vi "save channel config file.vi"(10 "Array":T1[](array[typedef]), 11 "file path":path) -> (3 "path":path)   [LabVIEW 2018]
uses:
  type defs/channelControl.ctl
  RT/Type Defs/channelScalingTypes.ctl
  RT/Type Defs/scalingMethods.ctl
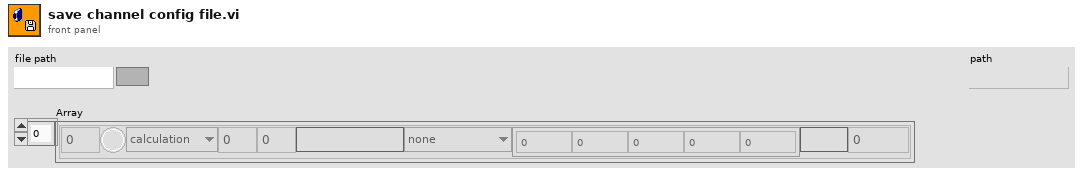
[diagram p1: front panel]
types:
  T1 = typedef "channelControl.ctl" = cluster{"index":u16, "active":bool, "channelType":T2, "module":u16, "terminal":u16, "channelName":string, "scalingMethod":T3, "scalingParameters":dbl[], "scaledUnits":string, "tempOffset":dbl}
  T2 = typedef "channelScalingTypes.ctl" = enum16{"calculation", "measurement", "scanivalve", "output", "digital"}
  T3 = typedef "scalingMethods.ctl" = enum16{"none", "linear", "thermocouple", "polynomial", "encoder", "RTD"}
  T4 = enum16{"open", "replace", "create", "open or create", "replace or create", "replace or create with confirmation"}
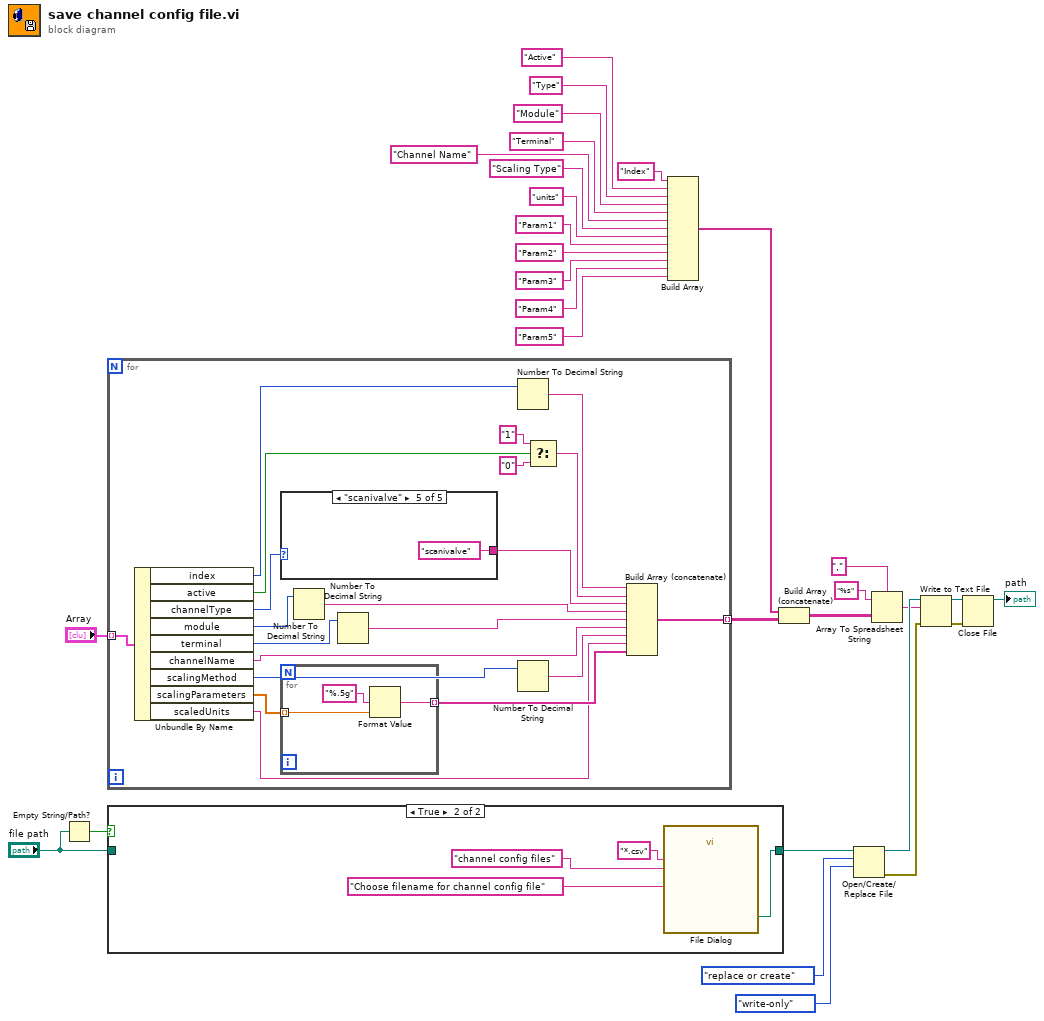
[diagram p0: block diagram]
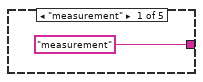
[diagram p3: hidden frame]
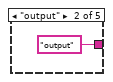
[diagram p4: hidden frame]
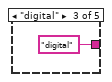
[diagram p5: hidden frame]
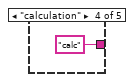
[diagram p6: hidden frame]
diagram:
  n1 = Empty String/Path?(string/path="file path") -> (empty?=w4:bool)
  n2 = for {
    tunnel: "Array" -> [w50] mode=indexing
    tunnel: [w38] -> w19 mode=indexing
    n3 = Unbundle By Name(w50) -> ("index"=w49:u16, "active"=w46:bool, "channelType"=w45:T2, "module"=w34:u16, "terminal"=w33:u16, "channelName"=w39:string, "scalingMethod"=w44:T3, "scalingParameters"=w43:dbl[], "scaledUnits"=w35:string)
    n4 = case shown="\"scanivalve\"" w45 {
      tunnel: ["measurement" ("f") "output" ("f") "digital" ("f") "calc" ("f") "scanivalve" ("f")] -> w40
      frame "measurement" {
      }
      frame "output" {
      }
      frame "digital" {
      }
      frame "calculation" {
      }
      frame "scanivalve" {
      }
    }
    n5 = for {
      tunnel: w43 -> [w53] mode=indexing
      tunnel: [w51] -> w37 mode=indexing
      n6 = Format Value(format string="%.5g", value (0)=w53) -> (output string=w51:string)  [unwired: 1 in]
    }
    n7 = Number To Decimal String(number=w34) -> (decimal integer string=w32:string)  [unwired: 1 in]
    n8 = Number To Decimal String(number=w33) -> (decimal integer string=w31:string)  [unwired: 1 in]
    n9 = Number To Decimal String(number=w49) -> (decimal integer string=w42:string)  [unwired: 1 in]
    n10 = Number To Decimal String(number=w44) -> (decimal integer string=w36:string)  [unwired: 1 in]
    n11 = Select(t="1", s=w46, f="0") -> (s? t:f=w41:string)
    n12 = Build Array (concatenate)(w42, w41, w40, w32, w31, w39, w36, w35, w37) -> (w38:string[])
  }
  n13 = case shown="True" w4 {
    tunnel: [w59 w62] -> w2
    tunnel: "file path" -> [w59 _]
    frame False {
    }
    frame True {
      n14 = call "File Dialog"("prompt"="Choose filename for channel config file", "pattern (all files)"="*.csv" ("pattern label"), "pattern label"="channel config files") -> ("selected path"=w62:path)  [unwired: 9 in, 3 out]
    }
  }
  n15 = Build Array("Index" ("t"), "Active" ("t"), "Type" ("t"), "Module" ("t"), "Terminal" ("t"), "Channel Name" ("t"), "Scaling Type" ("t"), "units" ("t"), "Param1" ("t"), "Param2" ("t"), "Param3" ("t"), "Param4" ("t"), "Param5" ("t")) -> (w18:string[])
  n16 = Build Array (concatenate)(w18, w19) -> (w29:string[][])
  n17 = Open/Create/Replace File(file path (use dialog)=w2, operation (0:open)=T4."replace or create", access (0:read/write)=enum16{"read/write", "read-only", "write-only"}."write-only") -> (refnum out=w23:refnum<file>, error out=w24:errorcluster)  [unwired: 3 in, 1 out]
  n18 = Array To Spreadsheet String(delimiter (Tab)=",", array=w29, 3:"%s" ("format string")) -> (spreadsheet string=w22:string)
  n19 = Write to Text File(file (use dialog)=w23, text=w22, error in=w24) -> (refnum out=w20:refnum<file>, error out=w21:errorcluster)  [unwired: 1 in, 1 out]
  n20 = Close File(refnum=w20, error in=w21) -> (path=→"path":path)  [unwired: 1 out]
